vi "ZigZagSkill.vi"(6 "ZigZag Number":u16, 8 "error in (no error)":errorcluster, 9 "Robot":refnum<class "Robot.lvclass">, 10 "Game in":refnum<class "Game.lvclass">, 11 "ZigZagSkill in":refnum<class "ZigZagSkill.lvclass">) -> (0 "error out":errorcluster, 1 "Game out":refnum<class "Game.lvclass">, 2 "Robot out":refnum<class "Robot.lvclass">, 3 "ZigZagSkill out":refnum<class "ZigZagSkill.lvclass">)   [LabVIEW 2018, in "ZigZagSkill.lvclass"]
uses:
  ZigZagSkill.lvclass
  Game_class/Game.lvclass
  Robot_class/Robot.lvclass
  Game_class/Game.lvclass/Game.ctl
  Utilities_class/Utilities.lvclass
  Object_class/Object.lvclass/Object.ctl
  Robot_class/Robot.lvclass/Robot.ctl
  Parameters_class/Parameters.lvclass/Parameters.ctl
  Object_class/Read x.vi
  Object_class/Read y.vi
  Robot_class/Read orientation.vi
  Game_class/Read Parameters.lvclass.vi
  Parameters_class/Read Angle.vi
  Robot_class/Write dest_x.vi
  Robot_class/Write dest_y.vi
  Robot_class/Write dest_orientation.vi
  Parameters_class/Parameters.lvclass
panel:
  out "element":cluster{"x":dbl, "y":dbl, "Angle":dbl}
  out "output array":bool[](array[boolean])
  in  "Change point by ID":bool[](array[boolean])
  out "Enable Change point":bool
  in  "Gravando":bool
  in  "file path (use dialog)":path=path "C:/temp/chutes.csv"
  in  "Time Target (s)":dbl=1.0
  out "Elapsed Time (s)":dbl
  in  "polar tolerance":dbl=50.0 format="%#_13g"
  in  "?":bool=TRUE
  in  "square tolerance":dbl=50.0 format="%#_13g"
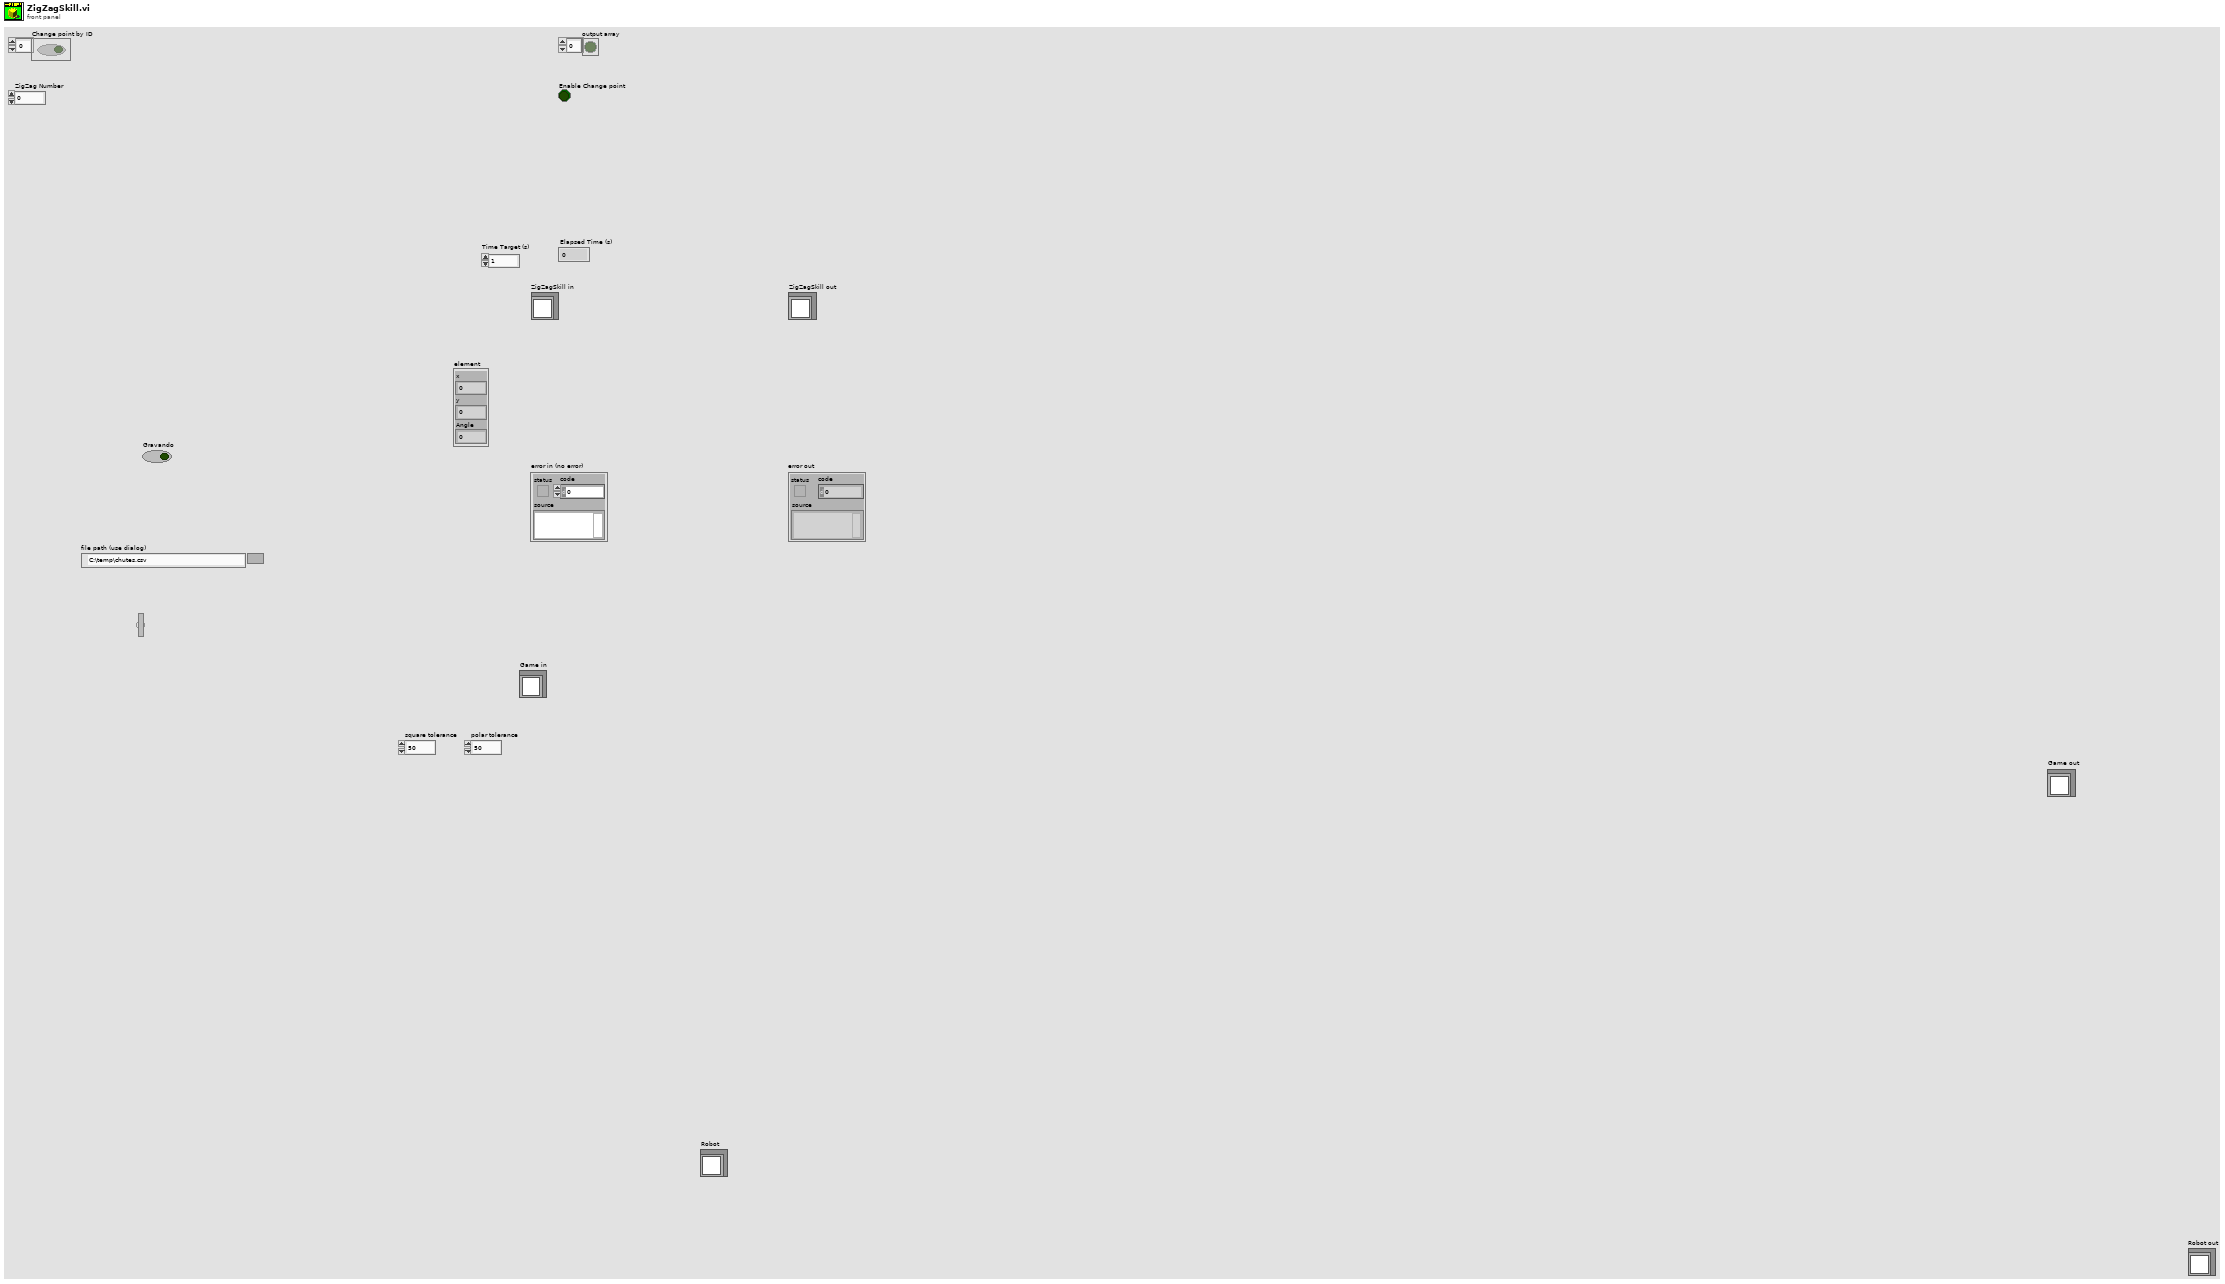
[diagram p1: front panel]
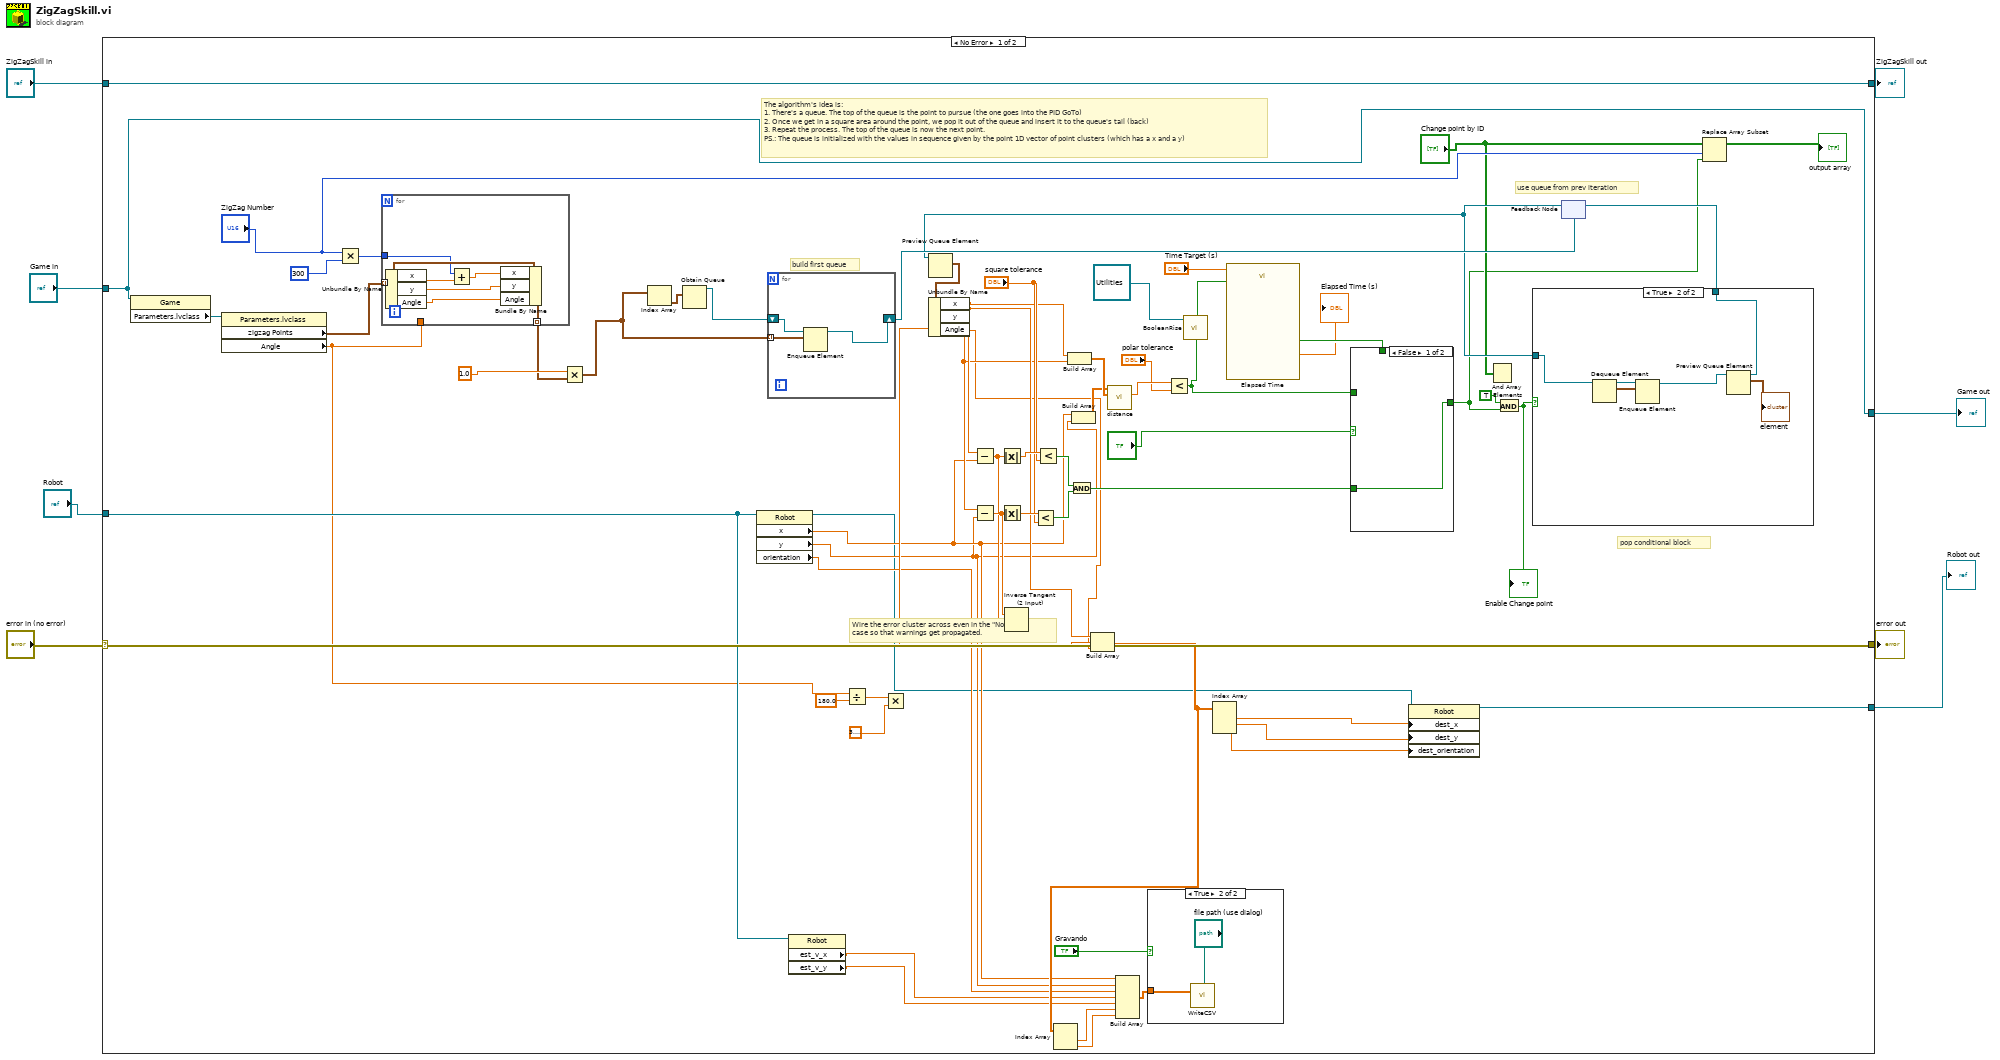
[diagram p0: block diagram]
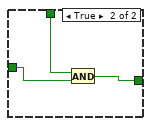
[diagram p3: hidden frame]
diagram:
  n1 = case shown="No Error" "error in (no error)" {
    selector: "error in (no error)" -> [w71 w99]
    tunnel: [w71 w99] -> w7
    tunnel: [w72 w98] -> w5
    tunnel: "ZigZagSkill in" -> [w72 w98]
    tunnel: "Game in" -> [w13 w96]
    tunnel: "Robot" -> [w14 w97]
    tunnel: [w13 w96] -> w2
    tunnel: [w12 w97] -> w1
    frame No Error {
      # "pop conditional block"
      # "use queue from prev iteration"
      # "The algorithm's idea is:\n1. There's a queue. The top of the queue is the point to pursue (the one goes into the PID GoTo)\n2. Once we get in a square area around the point, we pop it out of the queue and insert it to the queue's tail (back)\n3. Repeat the process. The top of the queue is now the next point.\nPS.: The queue is initialized with the values in sequence given by the point 1D vector of point clusters (which has a x and a y)"
      # "build first queue"
      # "Wire the error cluster across even in the \"No Error\"\ncase so that warnings get propagated."
      n2 = property class="Game"(reference=w13) -> ("Parameters.lvclass"=w26:refnum<class "Parameters.lvclass">)  [unwired: 1 in, 2 out]
      n3 = property class="Parameters.lvclass"(reference=w26) -> ("zigzag Points"=w25:cluster{"x":dbl, "y":dbl, "Angle":dbl}[], "Angle"=w10:dbl)  [unwired: 1 in, 2 out]
      n4 = Multiply(x="ZigZag Number", y=u16 300) -> (x*y=w33:u16)
      n5 = for {
        tunnel: w25 -> [w79] mode=indexing
        tunnel: w33 -> [w77]
        tunnel: [w74] -> w32 mode=indexing
        tunnel: w10 -> [_]
        n6 = Unbundle By Name(w79) -> ("x"=w78:dbl, "y"=w75:dbl, "Angle"=w73:dbl)
        n7 = Add(x=w77, y=w78) -> (x+y=w76:dbl)
        n8 = Bundle By Name(cluster=w79, "x"=w76, "y"=w75, "Angle"=w73) -> (w74:cluster{"x":dbl, "y":dbl, "Angle":dbl})
      }
      n9 = Multiply(x=1.0, y=w32) -> (x*y=w45:cluster{"x":dbl, "y":dbl, "Angle":dbl}[])
      n10 = Index Array(array=w45) -> (element=w70:cluster{"x":dbl, "y":dbl, "Angle":dbl})  [unwired: 1 in]
      n11 = Obtain Queue(element data type=w70) -> (queue out=w69:refnum<queue>)  [unwired: 4 in, 2 out]
      n12 = property class="Robot"(reference=w14) -> (reference out=w18:refnum<class "Robot.lvclass">, "x"=w24:dbl, "y"=w23:dbl, "orientation"=w22:dbl)  [unwired: 1 in, 1 out]
      n13 = for {
        tunnel: w45 -> [w94] mode=indexing
        shift-right: [w95] -> w62
        shift-left: w69 -> [w93]
        n14 = Enqueue Element(queue=w93, element=w94) -> (queue out=w95:refnum<queue>)  [unwired: 2 in, 2 out]
      }
      n15 = property class="Robot"(reference=w14) -> ("est_v_x"=w17:dbl, "est_v_y"=w16:dbl)  [unwired: 1 in, 2 out]
      n16 = Divide(x=w10, y=180.0) -> (x/y=w47:dbl)
      n17 = Multiply(x=w47, y=3.141592653589793) -> ()  [unwired: 1 out]
      n18 = Build Array(w24, w23) -> (w54:dbl[])
      n19 = And Array Elements(Boolean array="Change point by ID") -> ()  [unwired: 1 out]
      n20 = feedback #1(w62) -> (w61:refnum<queue>)
      n21 = Preview Queue Element(queue=w61) -> (element=w68:cluster{"x":dbl, "y":dbl, "Angle":dbl})  [unwired: 2 in, 3 out]
      n22 = Unbundle By Name(w68) -> ("x"=w57:dbl, "y"=w56:dbl, "Angle"=w9:dbl)
      n23 = Subtract(x=w57, y=w24) -> (x-y=w59:dbl)
      n24 = Subtract(x=w56, y=w23) -> (x-y=w60:dbl)
      n25 = Absolute Value(x=w59) -> (abs(x)=w67:dbl)
      n26 = Absolute Value(x=w60) -> (abs(x)=w66:dbl)
      n27 = Inverse Tangent (2 Input)(1:w59, 2:w60) -> ()  [unwired: 1 out]
      n28 = Less?(x=w66, y="square tolerance") -> (x < y?=w63:bool)
      n29 = Less?(x=w67, y="square tolerance") -> (x < y?=w64:bool)
      n30 = Build Array(w57, w56) -> (w55:dbl[])
      n31 = And(x=w64, y=w63) -> (x .and. y?=w50:bool)
      n32 = Build Array(w57, w56, w9) -> (w37:dbl[])
      n33 = Index Array(array=w37) -> (element #1=w36:dbl, element #2=w35:dbl)  [unwired: 2 in]
      n34 = call "distance.vi"("P1"=w55, "P2"=w54) -> ("Dist P1P2"=w52:dbl)  [unwired: 9 in]
      n35 = Build Array(w24, w23, w22, w17, w16, w36, w35) -> (w39:dbl[])
      n36 = case shown="True" "Gravando" {
        tunnel: w39 -> [_ w80]
        frame False {
        }
        frame True {
          n37 = call "WriteCSV.vi"("array"=w80, "file path (use dialog)"="file path (use dialog)") -> ()  [unwired: 10 in]
        }
      }
      n38 = Less?(x=w52, y="polar tolerance") -> (x < y?=w42:bool)
      n39 = call "BooleanRise.vi"("Boolean in"=w42, "Utilities in"=refnum<class "Utilities.lvclass"> refnum) -> ("Boolean"=w41:bool)  [unwired: 7 in, 2 out]
      n40 = Index Array(array=w37) -> (element #1=w21:dbl, element #2=w20:dbl, element #3=w19:dbl)  [unwired: 3 in]
      n41 = call "Elapsed Time"("Time Target (s)"="Time Target (s)", "Reset"=w41) -> ("Elapsed Time (s)"=→"Elapsed Time (s)":dbl, "Time has Elapsed"=w44:bool)  [unwired: 10 in, 6 out]
      n42 = case shown="False" "?" {
        tunnel: w42 -> [_ w85]
        tunnel: [w82 w84] -> w27
        tunnel: w50 -> [w82 _]
        tunnel: w44 -> [_ w83]
        frame False {
        }
        frame True {
          n43 = And(x=w83, y=w85) -> (x .and. y?=w84:bool)
        }
      }
      n44 = property class="Robot"(reference=w18, "dest_x"=w21, "dest_y"=w20, "dest_orientation"=w19) -> (reference out=w12:refnum<class "Robot.lvclass">)  [unwired: 1 in, 1 out]
      n45 = And(x=TRUE, y=w27) -> (x .and. y?=w28:bool)
      "Enable Change point" <- w28
      n46 = case shown="True" w28 {
        tunnel: w61 -> [w86 w90]
        tunnel: [w86 w88] -> w58
        frame False {
        }
        frame True {
          n47 = Dequeue Element(queue=w90) -> (queue out=w91:refnum<queue>, element=w92:cluster{"x":dbl, "y":dbl, "Angle":dbl})  [unwired: 2 in, 2 out]
          n48 = Enqueue Element(queue=w91, element=w92) -> (queue out=w89:refnum<queue>)  [unwired: 2 in, 2 out]
          n49 = Preview Queue Element(queue=w89) -> (queue out=w88:refnum<queue>, element=→"element":cluster{"x":dbl, "y":dbl, "Angle":dbl})  [unwired: 2 in, 2 out]
        }
      }
      n50 = feedback-in #1(w58) -> ()
      n51 = Replace Array Subset(array="Change point by ID", new element=w27, index="ZigZag Number") -> (→"output array":bool[])
    }
    frame Error {
    }
  }
  "error out" <- w7
  "ZigZagSkill out" <- w5
  "Game out" <- w2
  "Robot out" <- w1
